vi "i2c_sequence.vi"(6 "Bus":u8, 8 "error in":errorcluster, 9 "Sequence number":u8, 11 "I2C interface":T1) -> (0 "error out":errorcluster, 1 "Empty Elements Remaining":u32)   [LabVIEW 2014]
uses:
  i2c_interface.ctl
  fpga_reference.ctl
  Common/i2c_command.ctl
  <vilib>/Utility/error.llb/Error Cluster From Error Code.vi
  <vilib>/rvi/errors/niLvFpgaAdjustHostInterfaceError.vi
  <vilib>/rvi/interface/nirviMethod/nirviMethod.xnode
  FPGA Bitfiles/i2cmuxdemux.lvbitx
  <vilib>/FPGAPlugInAG/PCIe-7842R/niLvFpga_WriteFifo_PCIe-7842R.vi
  <vilib>/rvi/errors/niLvFpgaMergeErrorWithErrorCode.vi
panel:
  # "Send a wait_trigger command to the specified I2C bus.  If the FIFO is full then this VI will block until the data can be accepted."
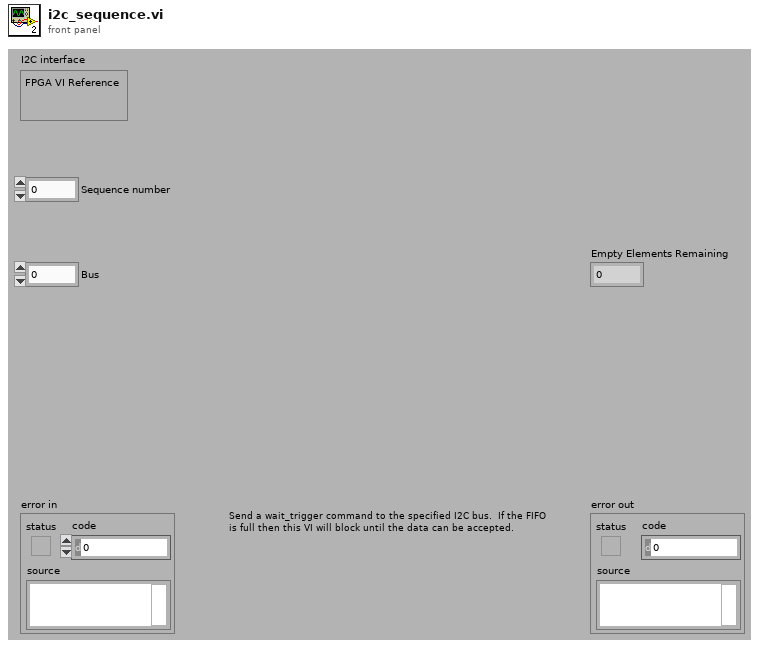
[diagram p1: front panel]
types:
  T1 = typedef "i2c_interface.ctl" = cluster{"FPGA VI Reference":T2}
  T2 = typedef "fpga_reference.ctl" = refnum<k20>
  T3 = typedef "i2c_command.ctl" = enum8{"invalid", "start_write", "start_read", "stop", "sequence"}
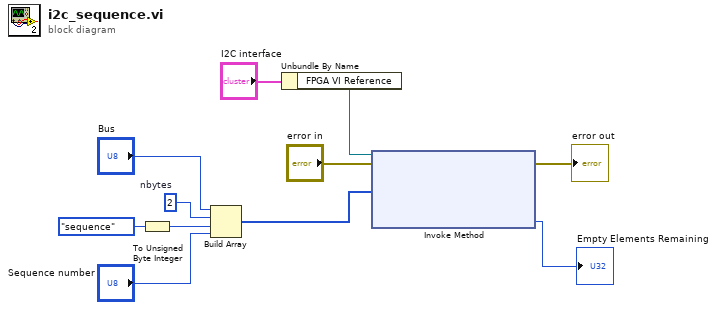
[diagram p0: block diagram]
diagram:
  w1 = u8 2  # nbytes
  n1 = To Unsigned Byte Integer(number=i2c_command."sequence" ("Command")) -> (unsigned 8bit integer=w5:u8)
  n2 = Build Array("Bus", w1, w5, "Sequence number") -> (w7:u8[])
  n3 = Unbundle By Name("I2C interface") -> ("FPGA VI Reference"=w10:T2)
  n4 = xnode "Invoke Method"("FPGA VI Reference In"=w10, "error in"="error in", "Data"=w7) -> ("error out"=→"error out":errorcluster, "Empty Elements Remaining"=→"Empty Elements Remaining":u32)  [unwired: 1 in, 1 out]
